vi "WPI_IMU_ADIS16448_Get AHRS.vi"(8 "error in":errorcluster, 11 "ADI IMU Interrupt DevRef":T1={"ADI IMU DevRef"={"DevStatus"={"status"=FALSE, "code"=0, "source"=""}, "Handle"=0, "SPI Bus"=enum."SPI On-Board, CS0", "Device Found"=FALSE, "Device Ready"=FALSE, "Yaw Axis"=enum."Z", "AHRS Algorithm"=enum."Complementary", "Serial"=0, "Lot ID 2"=0, "Lot ID 1"=0, "Product ID"=0}, "InterruptRef"={"DevStatus"={"status"=FALSE, "code"=0, "source"=""}, "InterruptIndex"=enum."0"}}) -> (0 "error out":errorcluster, 1 "IMU AHRS Delta Out":cluster{"Pitch":dbl, "Roll":dbl, "Yaw":dbl}, 2 "IMU AHRS Out":cluster{"Pitch":dbl, "Roll":dbl, "Yaw":dbl}, 3 "ADI IMU Interrupt DevRef":T1={"ADI IMU DevRef"={"DevStatus"={"status"=FALSE, "code"=0, "source"=""}, "Handle"=0, "SPI Bus"=enum."SPI On-Board, CS0", "Device Found"=FALSE, "Device Ready"=FALSE, "Yaw Axis"=enum."Z", "AHRS Algorithm"=enum."Complementary", "Serial"=0, "Lot ID 2"=0, "Lot ID 1"=0, "Product ID"=0}, "InterruptRef"={"DevStatus"={"status"=FALSE, "code"=0, "source"=""}, "InterruptIndex"=enum."0"}}, 4 "Sensor Ready Out":bool)   [LabVIEW 2015, in "Apple Pi Gyro Library.lvlib" / "FRC_ADIS16448_IMU.lvlib"]
doc: "Read accumulated angles from the Analog Devices IMU MXP board. Requires the IMU_Loop VI to be running in Periodic Tasks."
uses:
  FRC_ADIS16448_IMU.lvlib
  WPI_IMU_ADIS16448_InterruptDevRef.ctl
  WPI_IMU_ADIS16448_IMUDevRef.ctl
  <vilib>/Rock Robotics/SystemInterfaces/spilib/spi_bus.ctl
  <vilib>/Rock Robotics/WPI/Interrupt/WPI_InterruptRef.ctl
  <vilib>/Rock Robotics/SystemInterfaces/Interrupt/FPGA_InterruptIndex.ctl
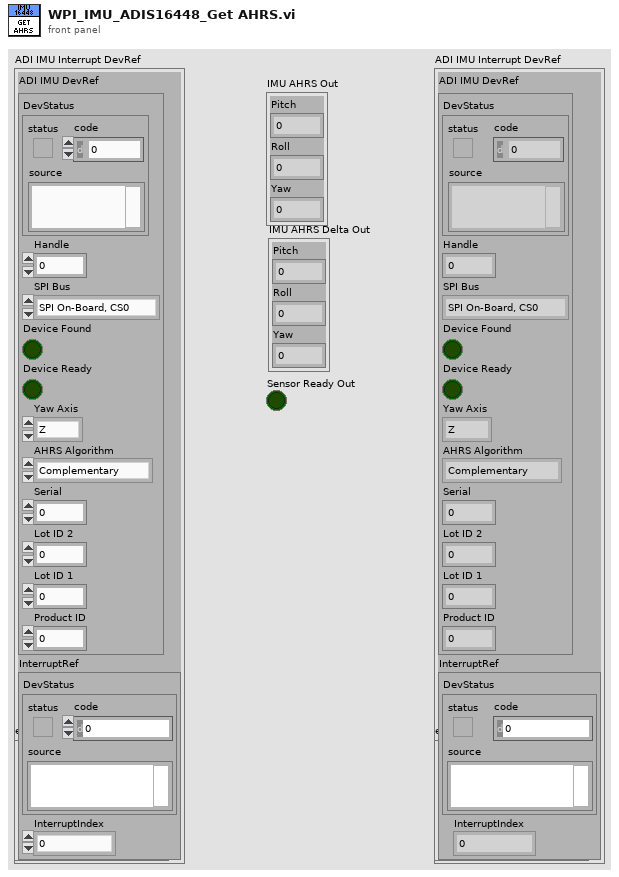
[diagram p1: front panel]
types:
  T1 = typedef "Apple Pi Gyro Library.lvlib/FRC_ADIS16448_IMU.lvlib/WPI_IMU_ADIS16448_InterruptDevRef.ctl" = cluster{"ADI IMU DevRef":T2, "InterruptRef":T4}
  T2 = typedef "Apple Pi Gyro Library.lvlib/FRC_ADIS16448_IMU.lvlib/WPI_IMU_ADIS16448_IMUDevRef.ctl" = cluster{"DevStatus":errorcluster, "Handle":i32, "SPI Bus":T3, "Device Found":bool, "Device Ready":bool, "Yaw Axis":enum16{"X", "Y", "Z"}, "AHRS Algorithm":enum16{"Complementary", "Madgwick"}, "Serial":u16, "Lot ID 2":u16, "Lot ID 1":u16, "Product ID":u16}
  T3 = typedef "spi_bus.ctl" = enum16{"SPI On-Board, CS0", "SPI On-Board, CS1", "SPI On-Board, CS2", "SPI On-Board, CS3", "SPI MXP", "Invalid"}
  T4 = typedef "WPI_InterruptRef.ctl" = cluster{"DevStatus":errorcluster, "InterruptIndex":T5}
  T5 = typedef "FPGA_InterruptIndex.ctl" = enum8{"0", "1", "2", "3", "4", "5", "6", "7", "Invalid"}
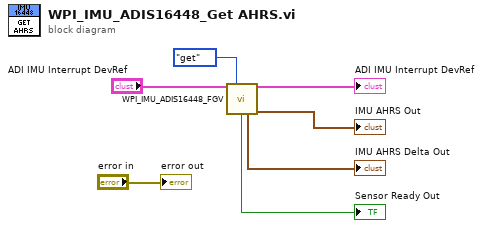
[diagram p0: block diagram]
diagram:
  n1 = call "WPI_IMU_ADIS16448_FGV.vi"("ADI IMU Interrupt DevRef"="ADI IMU Interrupt DevRef", "Operation"=enum16{"set", "get", "set reset"}."get") -> ("ADI IMU Interrupt DevRef Out"=→"ADI IMU Interrupt DevRef":T1, "Sensor Ready Out"=→"Sensor Ready Out":bool, "IMU AHRS Delta Out"=→"IMU AHRS Delta Out":cluster{"Pitch":dbl, "Roll":dbl, "Yaw":dbl}, "IMU AHRS Out"=→"IMU AHRS Out":cluster{"Pitch":dbl, "Roll":dbl, "Yaw":dbl})  [unwired: 7 in, 3 out]
  "error out" <- "error in"
